vi "HandleFitPars.vi"(6 "error in (no error)":errorcluster, 7 "Parameters in":T1(array[cluster]) {"value" format="%#.3f"}, 8 "Var params in":dbl[](array[numeric]), 9 "Task":T2(ring)=enum."Update") -> (0 "error out":errorcluster, 1 "Parameters out":T1(array[cluster]) {"value" format="%#.3f"}, 2 "Var params out":dbl[](array[numeric]), 3 "All params out":dbl[](array[numeric]), 4 "String":string)   [LabVIEW 2018]
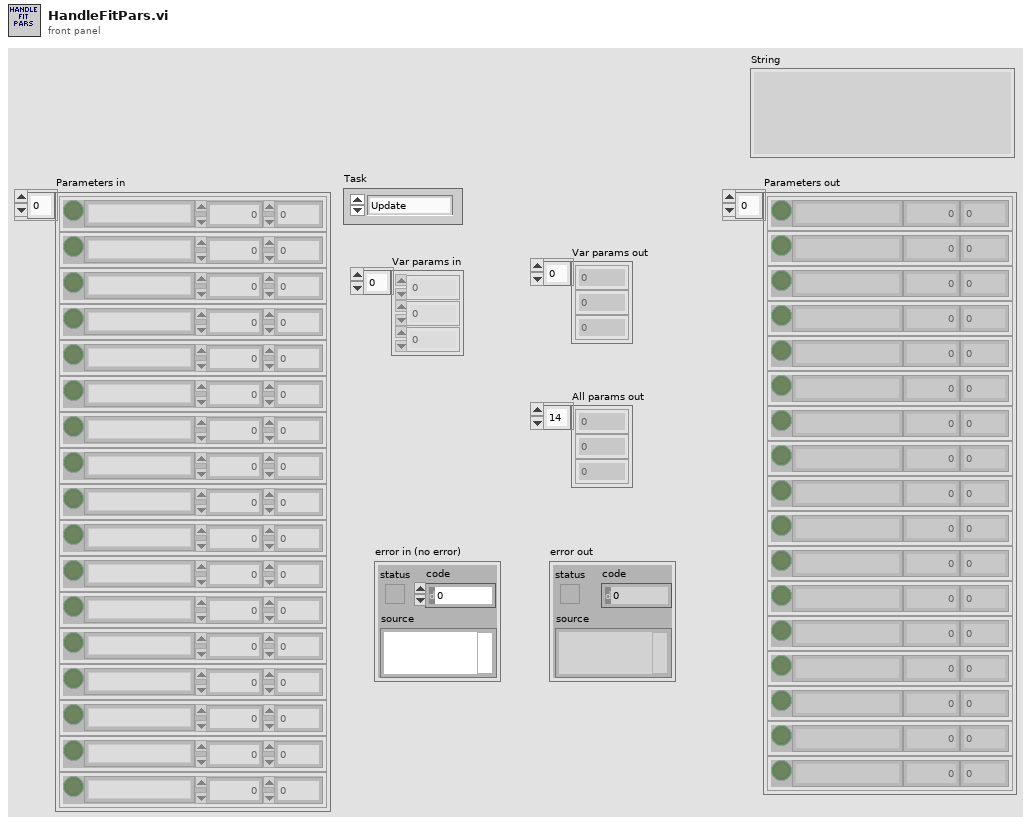
[diagram p1: front panel]
types:
  T1 = cluster{"fit":bool, "parname":string, "value":dbl, "SE":dbl}[]
  T2 = enum16{"Init", "Update", "Get", "Save", "Add SE", "To text"}
  T3 = cluster{"fit":bool, "parname":string, "value":dbl, "SE":dbl}
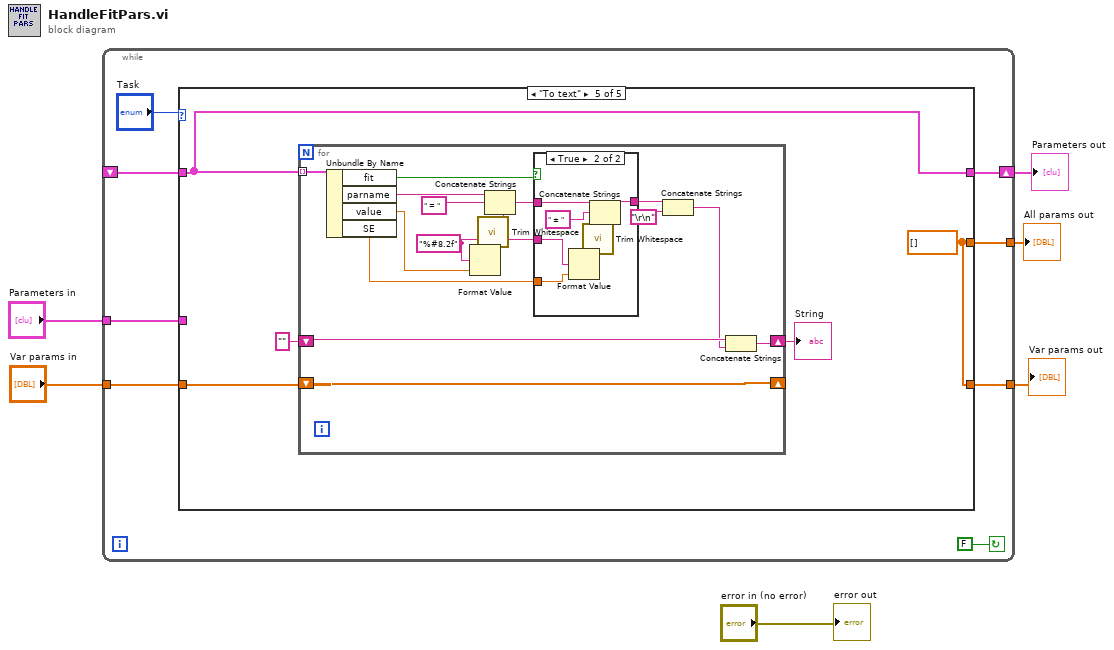
[diagram p0: block diagram]
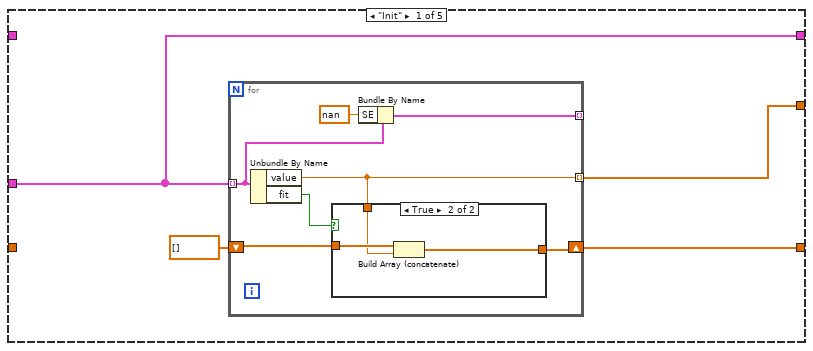
[diagram p2: hidden frame]
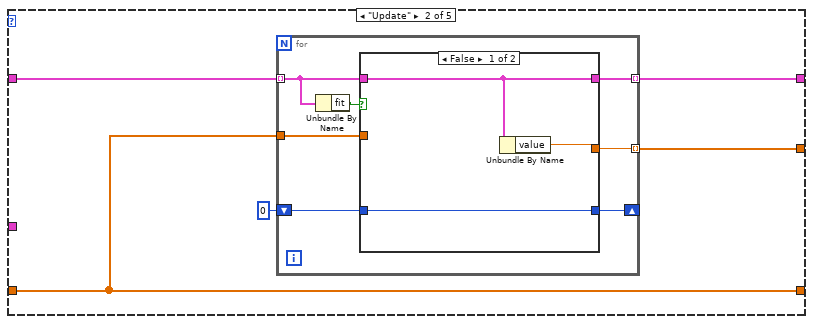
[diagram p4: hidden frame]
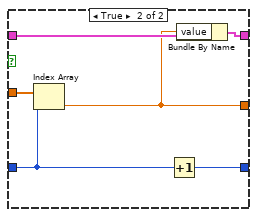
[diagram p5: hidden frame]
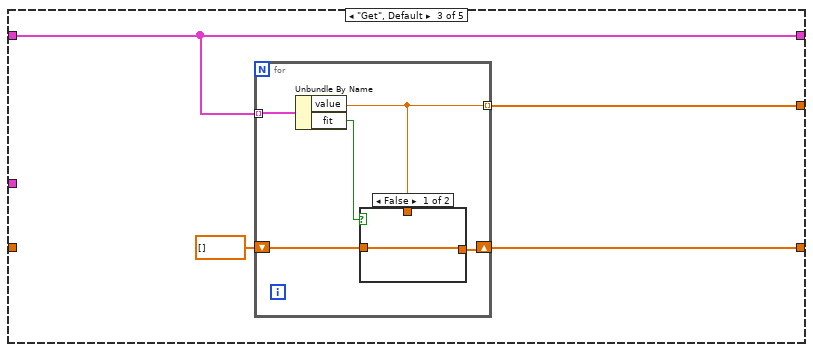
[diagram p6: hidden frame]
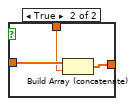
[diagram p7: hidden frame]
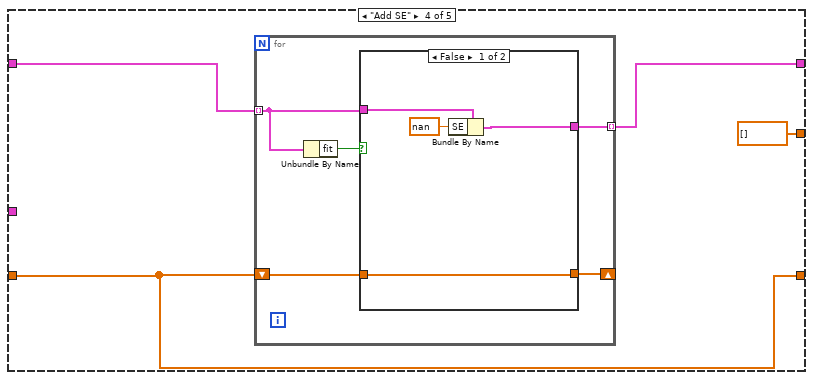
[diagram p8: hidden frame]
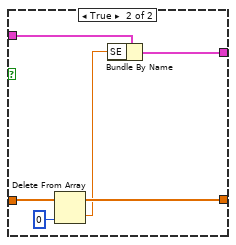
[diagram p9: hidden frame]
diagram:
  n1 = while {
    tunnel: [w11] -> w6
    tunnel: "Parameters in" -> [w10]
    shift-right: [w9] -> w2
    shift-left: _ -> [w8]
    tunnel: [w12] -> w5
    tunnel: "Var params in" -> [w7]
    stop <- FALSE continue-if-true
    n2 = case shown="\"To text\"" "Task" {
      tunnel: [w18 w31 w51 dbl[] [] w86] -> w12
      tunnel: [w16 w30 w53 w66 w86] -> w11
      tunnel: w10 -> [w15 _ _ _ _]
      tunnel: [w15 w32 w52 w65 w85] -> w9
      tunnel: w8 -> [_ w33 w52 w67 w85]
      tunnel: w7 -> [_ w30 _ w66 w87]
      frame "Init" {
        n3 = for {
          tunnel: w15 -> [w21] mode=indexing
          tunnel: [w24] -> w18 mode=indexing
          shift-right: [w23] -> w16
          shift-left: dbl[] [] -> [w25]
          tunnel: [w19] -> _ mode=indexing
          n4 = Unbundle By Name(w21) -> ("value"=w24:dbl, "fit"=w22:bool)
          n5 = case shown="True" w22 {
            tunnel: w25 -> [w26 w29]
            tunnel: w24 -> [_ w28]
            tunnel: [w26 w27] -> w23
            frame False {
            }
            frame True {
              n6 = Build Array (concatenate)(w29, w28) -> (w27:dbl[])
            }
          }
          n7 = Bundle By Name(cluster=w21, "SE"=nan) -> (w19:T3)
        }
      }
      frame "Update" {
        n8 = for {
          shift-right: [w40] -> _
          shift-left: 0 -> [w41]
          tunnel: w30 -> [w39]
          tunnel: w33 -> [w37] mode=indexing
          tunnel: [w36] -> w32 mode=indexing
          tunnel: [w35] -> w31 mode=indexing
          n9 = Unbundle By Name(w37) -> ("fit"=w38:bool)
          n10 = case shown="False" w38 {
            tunnel: w41 -> [w44 w50]
            tunnel: [w44 w49] -> w40
            tunnel: w39 -> [_ w48]
            tunnel: w37 -> [w43 w47]
            tunnel: [w43 w46] -> w36
            tunnel: [w42 w45] -> w35
            frame False {
              n11 = Unbundle By Name(w43) -> ("value"=w42:dbl)
            }
            frame True {
              n12 = Index Array(array=w48, index=w50) -> (element=w45:dbl)
              n13 = Increment(x=w50) -> (x+1=w49:i32)
              n14 = Bundle By Name(cluster=w47, "value"=w45) -> (w46:T3)
            }
          }
        }
      }
      frame "Get", Default {
        n15 = for {
          shift-right: [w55] -> w53
          shift-left: dbl[] [] -> [w59]
          tunnel: w52 -> [w58] mode=indexing
          tunnel: [w56] -> w51 mode=indexing
          n16 = Unbundle By Name(w58) -> ("value"=w56:dbl, "fit"=w57:bool)
          n17 = case shown="False" w57 {
            tunnel: w59 -> [w60 w63]
            tunnel: [w60 w62] -> w55
            tunnel: w56 -> [_ w61]
            frame False {
            }
            frame True {
              n18 = Build Array (concatenate)(w63, w61) -> (w62:dbl[])
            }
          }
        }
      }
      frame "Add SE" {
        n19 = for {
          tunnel: w67 -> [w71] mode=indexing
          shift-right: [w69] -> _
          shift-left: w66 -> [w70]
          tunnel: [w68] -> w65 mode=indexing
          n20 = Unbundle By Name(w71) -> ("fit"=w72:bool)
          n21 = case shown="False" w72 {
            tunnel: w71 -> [w76 w82]
            tunnel: w70 -> [w73 w81]
            tunnel: [w73 w79] -> w69
            tunnel: [w75 w77] -> w68
            frame False {
              n22 = Bundle By Name(cluster=w76, "SE"=nan) -> (w75:T3)
            }
            frame True {
              n23 = Delete From Array(array=w81, index=0) -> (deleted portion=w78:dbl, array with subset deleted=w79:dbl[])  [unwired: 1 in]
              n24 = Bundle By Name(cluster=w82, "SE"=w78) -> (w77:T3)
            }
          }
        }
      }
      frame "To text" {
        w86 = dbl[] []
        n25 = for {
          tunnel: w85 -> [w103] mode=indexing
          shift-right: [w102] -> _
          shift-left: w87 -> [w102]
          shift-right: [w94] -> w83
          shift-left: "" -> [w93]
          w97 = "%#8.2f" ("format string")
          n26 = Unbundle By Name(w103) -> ("fit"=w99:bool, "parname"=w101:string, "value"=w100:dbl, "SE"=w91:dbl)
          n27 = Format Value(format string=w97, value (0)=w100) -> (output string=w89:string)  [unwired: 1 in]
          n28 = call <vilib>:"Trim Whitespace.vi"("string"=w89) -> ("trimmed string"=w88:string)  [unwired: 1 in]
          n29 = Concatenate Strings(w101, " = " ("string"), w88) -> (w98:string)
          n30 = case shown="True" w99 {
            tunnel: [w104 w111] -> w96
            tunnel: w98 -> [w104 w110]
            tunnel: w97 -> [_ w108]
            tunnel: w91 -> [_ w107]
            frame False {
            }
            frame True {
              n31 = Format Value(format string=w108, value (0)=w107) -> (output string=w109:string)  [unwired: 1 in]
              n32 = call <vilib>:"Trim Whitespace.vi"("string"=w109) -> ("trimmed string"=w106:string)  [unwired: 1 in]
              n33 = Concatenate Strings(w110, " ± " ("*(type *) &x"), w106) -> (w111:string)
            }
          }
          n34 = Concatenate Strings(w96, "\r\n") -> (w92:string)
          n35 = Concatenate Strings(w93, w92) -> (w94:string)
        }
        "String" <- w83
      }
    }
  }
  "All params out" <- w5
  "Var params out" <- w6
  "Parameters out" <- w2
  "error out" <- "error in (no error)"
